vi "NXT Timer 2.vi"() -> (5 "Branched Timer Index":T1)   [LabVIEW 2010, in "timerExts.lvlib"]
uses:
  timerExts.lvlib
  Branched Timer.ctl
  <vilib>/NXT/Block Support/NXT_TimerIndex.ctl
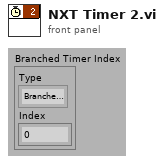
[diagram p1: front panel]
types:
  T1 = typedef "timerExts.lvlib/Branched Timer.ctl" = cluster{"Type":enum8{"Branched Timer", "NXT Timer"}, "Index":u16}
  T2 = typedef "NXT_TimerIndex.ctl" = u8
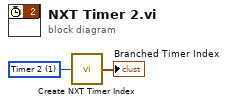
[diagram p0: block diagram]
diagram:
  w2 = T2 1 items=["Timer 1", "Timer 2", "Timer 3"] ("Timer (Timer 1)")
  n1 = call "Create NXT Timer Index.vi"("Timer (Timer 1)"=w2) -> ("Branched Timer Index"=→"Branched Timer Index":T1)
